vi "Any_limit_switch_active.vi"(6 "Echo Mode":i32, 8 "error in (no error)":errorcluster, 11 "VISA resource name":refnum<visa-resource-name>) -> (0 "error out":errorcluster={"status"=FALSE, "code"=1073676294, "source"="VISA Read in write_read.vi"}, 1 "limit switch cluster":T1, 2 "motor error cluster":T2, 3 "VISA ressource out":refnum<visa-resource-name>, 5 "Any Limit Switch?":bool)   [LabVIEW 2018]
uses:
  Surveillance/limit_switch_Cluster.ctl
panel:
  in  "limit switch cluster IN":T1
  in  "Error M 4":bool
  in  "Error M 3":bool
  in  "Error M 2":bool
  in  "Error M 1":bool
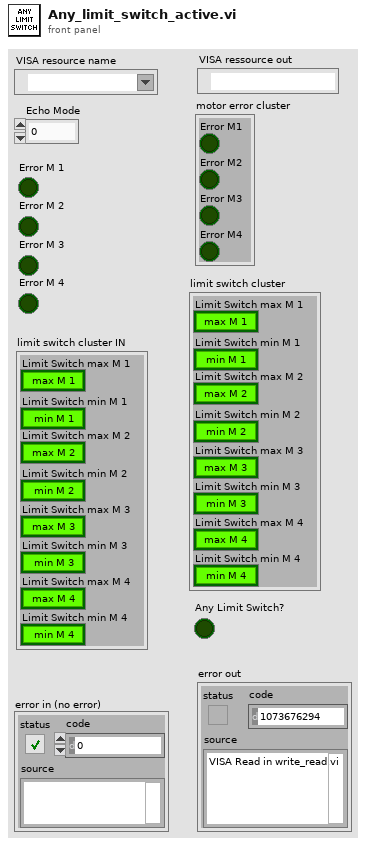
[diagram p1: front panel]
types:
  T1 = typedef "limit_switch_Cluster.ctl" = cluster{"Limit Switch max M 1":bool, "Limit Switch min M 1":bool, "Limit Switch max M 2":bool, "Limit Switch min M 2":bool, "Limit Switch max M 3":bool, "Limit Switch min M 3":bool, "Limit Switch max M 4":bool, "Limit Switch min M 4":bool}
  T2 = cluster{"Error M1":bool, "Error M2":bool, "Error M3":bool, "Error M4":bool}
  T3 = cluster{"Error M 1":bool, "Error M 2":bool, "Error M 3":bool, "Error M 4":bool}
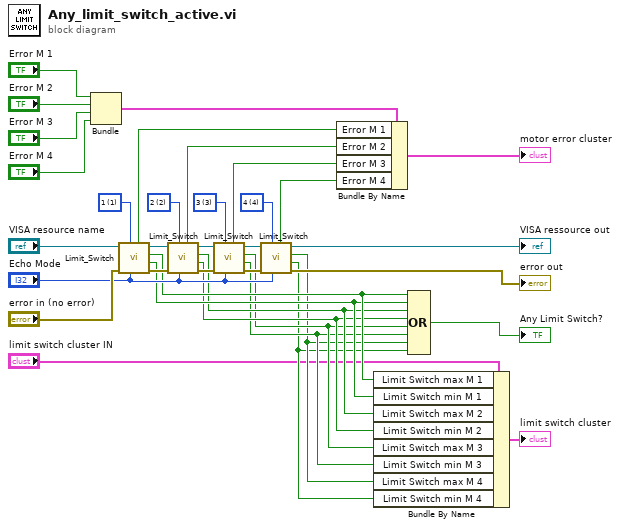
[diagram p0: block diagram]
diagram:
  w31 = u16 4 items=["none", "1", "2", "3", "4", "all"] ("Motor")
  w32 = u16 3 items=["none", "1", "2", "3", "4", "all"] ("Motor")
  w33 = u16 2 items=["none", "1", "2", "3", "4", "all"] ("Motor")
  w34 = u16 1 items=["none", "1", "2", "3", "4", "all"] ("Motor")
  n1 = Bundle("Error M 1"="Error M 1", "Error M 2"="Error M 2", "Error M 3"="Error M 3", "Error M 4"="Error M 4") -> (w13:T3)  [unwired: 1 in]
  n2 = call "Limit_Switch.vi"("Echo Mode"="Echo Mode", "Motor"=w34, "error in (no error)"="error in (no error)", "VISA resource name"="VISA resource name") -> ("error out"=w29:errorcluster, "Limit Switch min"=w9:bool, "Limit Switch max"=w10:bool, "VISA ressource out"=w30:refnum<visa-resource-name>, "Error?"=w21:bool)  [unwired: 3 in]
  n3 = call "Limit_Switch.vi"("Echo Mode"="Echo Mode", "Motor"=w33, "error in (no error)"=w29, "VISA resource name"=w30) -> ("error out"=w28:errorcluster, "Limit Switch min"=w7:bool, "Limit Switch max"=w8:bool, "VISA ressource out"=w27:refnum<visa-resource-name>, "Error?"=w20:bool)  [unwired: 3 in]
  n4 = call "Limit_Switch.vi"("Echo Mode"="Echo Mode", "Motor"=w32, "error in (no error)"=w28, "VISA resource name"=w27) -> ("error out"=w25:errorcluster, "Limit Switch min"=w5:bool, "Limit Switch max"=w6:bool, "VISA ressource out"=w26:refnum<visa-resource-name>, "Error?"=w19:bool)  [unwired: 3 in]
  n5 = call "Limit_Switch.vi"("Echo Mode"="Echo Mode", "Motor"=w31, "error in (no error)"=w25, "VISA resource name"=w26) -> ("error out"=→"error out":errorcluster, "Limit Switch min"=w3:bool, "Limit Switch max"=w4:bool, "VISA ressource out"=→"VISA ressource out":refnum<visa-resource-name>, "Error?"=w18:bool)  [unwired: 3 in]
  n6 = Bundle By Name(cluster=w13, "Error M 1"=w21, "Error M 2"=w20, "Error M 3"=w19, "Error M 4"=w18) -> (→"motor error cluster":T3)
  n7 = Bundle By Name(cluster="limit switch cluster IN", "Limit Switch max M 1"=w10, "Limit Switch min M 1"=w9, "Limit Switch max M 2"=w8, "Limit Switch min M 2"=w7, "Limit Switch max M 3"=w6, "Limit Switch min M 3"=w5, "Limit Switch max M 4"=w4, "Limit Switch min M 4"=w3) -> (→"limit switch cluster":T1)
  n8 = Compound Arithmetic op=OR(w10, w9, w8, w7, w6, w5, w4, w3) -> (→"Any Limit Switch?":bool)
